vi "FTW-Endpoint-CreateReader.vi"(0 "FTW-Endpoint-TCP In":refnum<class "FTW-Endpoint-TCP.lvclass">, 5 "Address":string, 9 "Timeout":i32=1000 format="%dmsec", 11 "error in":errorcluster) -> (4 "FTW-Endpoint-TCP Out":refnum<class "FTW-Endpoint-TCP.lvclass">, 6 "Actual Address":string, 15 "error out":errorcluster)   [LabVIEW 2013, in "FTW-Endpoint-TCP.lvclass"]
uses:
  FTW-Endpoint-TCP.lvclass
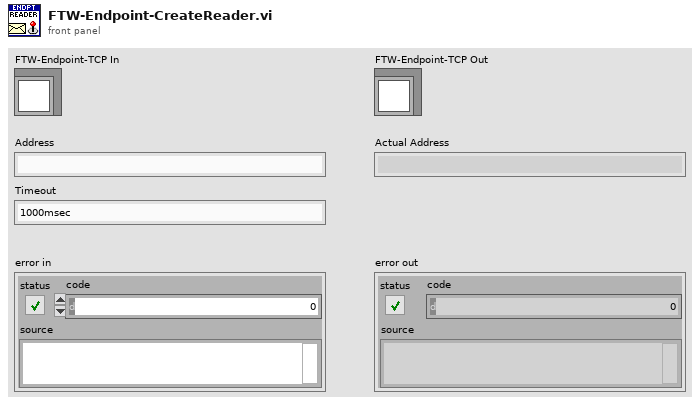
[diagram p1: front panel]
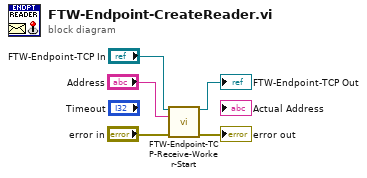
[diagram p0: block diagram]
diagram:
  n1 = call-dynamic "FTW-Endpoint-TCP-Receive-Worker-Start.vi"("FTW-Endpoint-TCP In"="FTW-Endpoint-TCP In", "Endpoint Address"="Address", "error in"="error in") -> ("FTW-Endpoint-TCP Out"=→"FTW-Endpoint-TCP Out":refnum<class "FTW-Endpoint-TCP.lvclass">, "error out"=→"error out":errorcluster)  [unwired: 11 in]
